vi "SpikeRejector.vi"(2 "Average Only (T)":bool, 3 "SigmaFactor":dbl format="%.2f", 5 "Input Array":dbl[][](array[numeric]) format="%.2f") -> (0 "Sigma Array":dbl[](array[numeric]), 1 "Final Array":dbl[](array[numeric]) format="%.2f")   [LabVIEW 2020]
doc: "This VI takes a 2D array input, with different rows representing different spectral shots and columns for different wavelegnths.\nAverage of all shots are computed and then filter out those falling out of the SigmaFactor range. The remaing ones are re-calculated for average.\n\nSuggested Sigma Factor is 1 (67% pass). Good values are between 0.5 and 2."
uses:
  <vilib>/Analysis/NI_AALBase.lvlib
panel:
  out "Waveform Graph":dbl[][](graph)
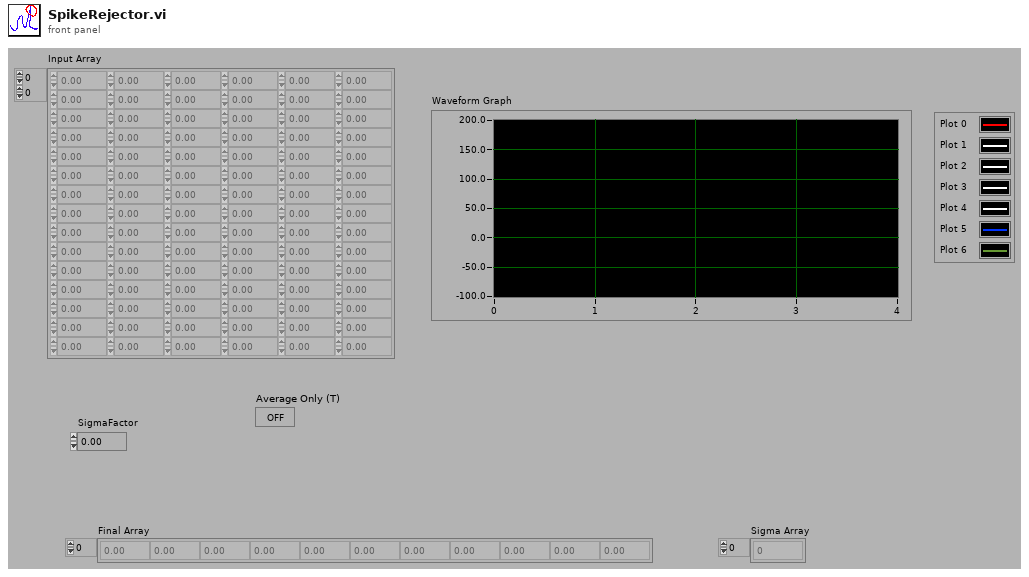
[diagram p1: front panel]
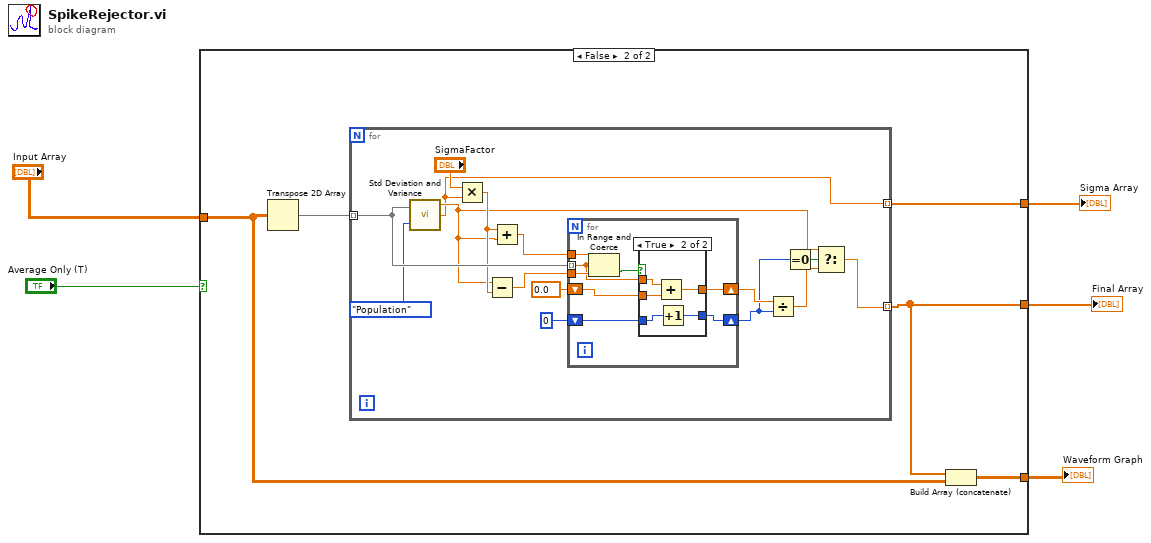
[diagram p0: block diagram]
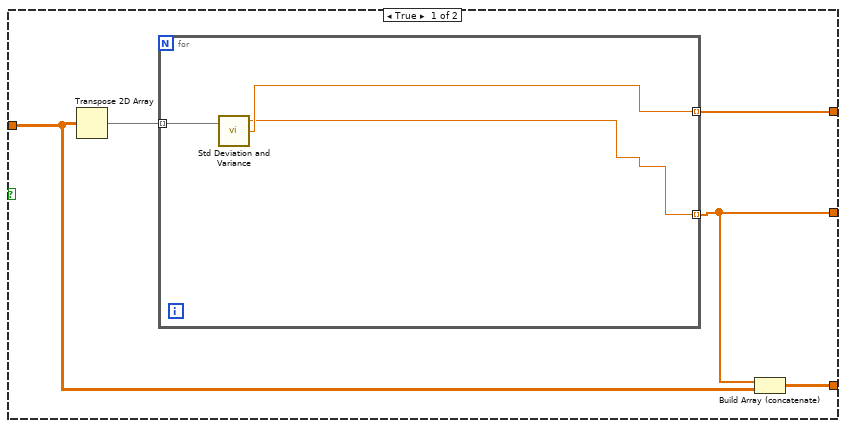
[diagram p2: hidden frame]
diagram:
  n1 = case shown="False" "Average Only (T)" {
    tunnel: [w10 w18] -> w5
    tunnel: [w9 w17] -> w4
    tunnel: "Input Array" -> [w7 w15]
    tunnel: [w6 w14] -> w3
    frame True {
      n2 = Transpose 2D Array(2D array=w7) -> (transposed array=w8:dbl[][])
      n3 = for {
        tunnel: w8 -> [w13] mode=indexing
        tunnel: [w11] -> w10 mode=indexing
        tunnel: [w12] -> w6 mode=indexing
        n4 = call <vilib>:"Std Deviation and Variance.vi"("X"=w13) -> ("mean"=w11:dbl, "standard deviation"=w12:dbl)  [unwired: 1 in, 1 out]
      }
      n5 = Build Array (concatenate)(w10, w7) -> (w9:dbl[][])
    }
    frame False {
      n6 = Transpose 2D Array(2D array=w15) -> (transposed array=w16:dbl[][])
      n7 = for {
        tunnel: w16 -> [w32] mode=indexing
        tunnel: [w21] -> w18 mode=indexing
        tunnel: [w19] -> w14 mode=indexing
        n8 = call <vilib>:"Std Deviation and Variance.vi"("X"=w32, "Weighting (Sample)"=enum16{"Sample", "Population"}."Population") -> ("mean"=w20:dbl, "standard deviation"=w19:dbl)  [unwired: 1 out]
        n9 = Multiply(x="SigmaFactor", y=w19) -> (x*y=w31:dbl)
        n10 = Subtract(x=w20, y=w31) -> (x-y=w30:dbl)
        n11 = Add(x=w31, y=w20) -> (x+y=w29:dbl)
        n12 = for {
          tunnel: w32 -> [w36] mode=indexing
          tunnel: w30 -> [w41]
          tunnel: w29 -> [w40]
          shift-right: [w38] -> w27
          shift-left: 0.0 -> [w37]
          shift-right: [w35] -> w23
          shift-left: u32 0 -> [w34]
          n13 = In Range and Coerce(upper limit=w40, x=w36, lower limit=w41) -> (In Range?=w39:bool)  [unwired: 1 out]
          n14 = case shown="True" w39 {
            tunnel: [w43 w48] -> w38
            tunnel: w37 -> [w43 w47]
            tunnel: w36 -> [_ w46]
            tunnel: [w42 w45] -> w35
            tunnel: w34 -> [w42 w44]
            frame False {
            }
            frame True {
              n15 = Add(x=w46, y=w47) -> (x+y=w48:dbl)
              n16 = Increment(x=w44) -> (x+1=w45:u32)
            }
          }
        }
        n17 = Divide(x=w27, y=w23) -> (x/y=w22:dbl)
        n18 = Equal To 0?(x=w23) -> (x = 0?=w24:bool)
        n19 = Select(t=w20, s=w24, f=w22) -> (s? t:f=w21:dbl)
      }
      n20 = Build Array (concatenate)(w18, w15) -> (w17:dbl[][])
    }
  }
  "Final Array" <- w5
  "Waveform Graph" <- w4
  "Sigma Array" <- w3
